vi "SelectTrial.vi"(1 "TargetsCluster":T1={"Start"={"Horiz"=0.0, "Vert"=0.0, "Radius"=0.5, "Hide"=FALSE}, "Pos1"={"Horiz"=4.25, "Vert"=0.0, "Radius"=0.5, "Hide"=FALSE}, "Pos2"={"Horiz"=4.25, "Vert"=2.5, "Radius"=0.5, "Hide"=FALSE}, "Pos3"={"Horiz"=0.0, "Vert"=2.5, "Radius"=0.5, "Hide"=FALSE}, "Pos4"={"Horiz"=-4.25, "Vert"=2.5, "Radius"=0.5, "Hide"=FALSE}, "Pos5"={"Horiz"=-4.25, "Vert"=0.0, "Radius"=0.5, "Hide"=FALSE}, "Pos6"={"Horiz"=-4.25, "Vert"=-2.5, "Radius"=0.5, "Hide"=FALSE}, "Pos7"={"Horiz"=0.0, "Vert"=-2.5, "Radius"=0.5, "Hide"=FALSE}, "Pos8"={"Horiz"=4.25, "Vert"=-2.5, "Radius"=0.5, "Hide"=FALSE}} caption="Target Positions" {"Pos8"."Radius" min=-5.0 max=5.0 step=0.5 format="%.2f"; "Pos8"."Vert" min=-5.0 max=5.0 step=0.5 format="%.2f"; "Pos8"."Horiz" min=-5.0 max=5.0 step=0.25 format="%.2f"; "Pos7"."Radius" min=-5.0 max=5.0 step=0.5 format="%.2f"; "Pos7"."Vert" min=-5.0 max=5.0 step=0.5 format="%.2f"; "Pos7"."Horiz" min=-5.0 max=5.0 step=0.25 format="%.2f"; "Pos6"."Radius" min=-5.0 max=5.0 step=0.5 format="%.2f"; "Pos6"."Vert" min=-5.0 max=5.0 step=0.5 format="%.2f"; "Pos6"."Horiz" min=-5.0 max=5.0 step=0.25 format="%.2f"; "Pos5"."Radius" min=-5.0 max=5.0 step=0.5 format="%.2f"; "Pos5"."Vert" min=-5.0 max=5.0 step=0.5 format="%.2f"; "Pos5"."Horiz" min=-5.0 max=5.0 step=0.25 format="%.2f"; "Pos4"."Radius" min=-5.0 max=5.0 step=0.5 format="%.2f"; "Pos4"."Vert" min=-5.0 max=5.0 step=0.5 format="%.2f"; "Pos4"."Horiz" min=-5.0 max=5.0 step=0.25 format="%.2f"; "Pos3"."Radius" min=-5.0 max=5.0 step=0.5 format="%.2f"; "Pos3"."Vert" min=-5.0 max=5.0 step=0.5 format="%.2f"; "Pos3"."Horiz" min=-5.0 max=5.0 step=0.25 format="%.2f"; "Pos2"."Radius" min=-5.0 max=5.0 step=0.5 format="%.2f"; "Pos2"."Vert" min=-5.0 max=5.0 step=0.5 format="%.2f"; "Pos2"."Horiz" min=-5.0 max=5.0 step=0.25 format="%.2f"; "Pos1"."Radius" min=-5.0 max=5.0 step=0.5 format="%.2f"; "Pos1"."Vert" min=-5.0 max=5.0 step=0.5 format="%.2f"; "Pos1"."Horiz" min=-5.0 max=5.0 step=0.25 format="%.2f"; "Start"."Radius" min=-5.0 max=5.0 step=0.5 format="%.2f"; "Start"."Vert" min=-5.0 max=5.0 step=0.5 format="%.2f"; "Start"."Horiz" min=-5.0 max=5.0 step=0.25 format="%.2f"}) -> (0 "TrialType":i32)   [LabVIEW 2010]
uses:
  <vilib>/imath/engines/lvmath2/RunTimeEngine/ErrorHandling/NIMS_Finalize Error.vi
  <vilib>/imath/engines/lvmath2/RunTimeEngine/RangeToken/NIMS_Range_R2.vi
  <vilib>/imath/engines/lvmath2/RunTimeEngine/VariableToken/Read/NIMS_Get Elements - RV(_) - Check.vi
  <instcachedir>/0/NIMS_Get Elements - RV(_) - Check_1F6F8656162345078B1D4DC9877DFAE9.lvgen/NIMS_Get Elements - RV(_) - Check_1F6F8656162345078B1D4DC9877DFAE9_003.vi
  <vilib>/imath/engines/lvmath2/RunTimeEngine/BuiltInFunctions/findnz/NIMS_[1o]_findnz(GRowV).vi
  <instcachedir>/0/NIMS_[1o]_findnz(GRowV)_005A6E28988F485CA06F579662DA62C7.lvgen/NIMS_[1o]_findnz(GRowV)_005A6E28988F485CA06F579662DA62C7_000.vi
  <vilib>/imathl/engines/lvmath/Functions/Error Handling/Create Error.vi
  <vilib>/imath/engines/lvmath2/RunTimeEngine/BuiltInFunctions/is_empty/NIMS_is_empty(GV).vi
  <instcachedir>/0/NIMS_is_empty(GV)_FC7E7C3D9544432CB6AA2416ADCF6D56.lvgen/NIMS_is_empty(GV)_FC7E7C3D9544432CB6AA2416ADCF6D56_000.vi
  <vilib>/imath/engines/lvmath2/RunTimeEngine/NodeEndStatement/NIMS_NodeEndStatement_Output.vi
  <instcachedir>/0/NIMS_NodeEndStatement_Output_53EC0D466D134D7ABD903AC30B43404B.lvgen/NIMS_NodeEndStatement_Output_53EC0D466D134D7ABD903AC30B43404B_010.vi
  <vilib>/imath/engines/lvmath2/RunTimeEngine/BuiltInFunctions/length/NIMS_length(GV).vi
  <instcachedir>/0/NIMS_length(GV)_08A3D13377FD4E4B96F5795FBF3698FA.lvgen/NIMS_length(GV)_08A3D13377FD4E4B96F5795FBF3698FA_002.vi
  <vilib>/imath/engines/lvmath2/RunTimeEngine/BuiltInFunctions/rand/NIMS_rand().vi
  <vilib>/imath/engines/lvmath2/RunTimeEngine/BuiltInFunctions/fix/NIMS_fix(DBL-S).vi
  <vilib>/imath/engines/lvmath2/RunTimeEngine/VariableToken/Read/NIMS_Get Elements - RV(_) - Check(_).vi
  <instcachedir>/0/NIMS_Get Elements - RV(_) - Check(_)_260A45C9C4AF472A8F32F86A1BEF7DEE.lvgen/NIMS_Get Elements - RV(_) - Check(_)_260A45C9C4AF472A8F32F86A1BEF7DEE_000.vi
  <vilib>/imath/engines/lvmath2/RunTimeEngine/ErrorHandling/NIMS_Create Error From Enums.vi
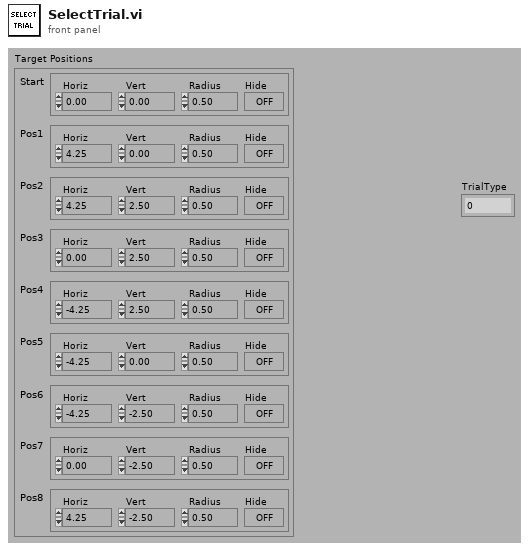
[diagram p1: front panel]
types:
  T1 = cluster{"Start":cluster{"Horiz":dbl, "Vert":dbl, "Radius":dbl, "Hide":bool}, "Pos1":cluster{"Horiz":dbl, "Vert":dbl, "Radius":dbl, "Hide":bool}, "Pos2":cluster{"Horiz":dbl, "Vert":dbl, "Radius":dbl, "Hide":bool}, "Pos3":cluster{"Horiz":dbl, "Vert":dbl, "Radius":dbl, "Hide":bool}, "Pos4":cluster{"Horiz":dbl, "Vert":dbl, "Radius":dbl, "Hide":bool}, "Pos5":cluster{"Horiz":dbl, "Vert":dbl, "Radius":dbl, "Hide":bool}, "Pos6":cluster{"Horiz":dbl, "Vert":dbl, "Radius":dbl, "Hide":bool}, "Pos7":cluster{"Horiz":dbl, "Vert":dbl, "Radius":dbl, "Hide":bool}, "Pos8":cluster{"Horiz":dbl, "Vert":dbl, "Radius":dbl, "Hide":bool}}
  T2 = cluster{"Horiz":dbl, "Vert":dbl, "Radius":dbl, "Hide":bool}[]
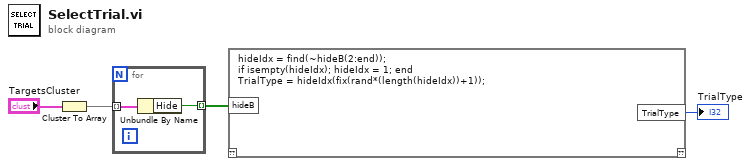
[diagram p0: block diagram]
diagram:
  n1 = Cluster To Array(cluster="TargetsCluster") -> (array=w4:T2)
  n2 = for {
    tunnel: w4 -> [w6] mode=indexing
    tunnel: [w5] -> w2 mode=indexing
    n3 = Unbundle By Name(w6) -> ("Hide"=w5:bool)
  }
  n4 = mathscript code="hideIdx = find(~hideB(2:end));\nif isempty(hideIdx); hideIdx = 1; end\nTrialType = hideIdx(fix(rand*(length(hideIdx))+1));"("hideB"=w2) -> ("TrialType"=→"TrialType":i32)  [unwired: 1 in, 1 out]
